vi "Day 3.vi"() -> ()   [LabVIEW 2020]
uses:
  40740d06-73ee-45d0-88f6-0b9eb97e4559.vi
  6b01a3fd-33d4-4bb7-9d17-933a35c8bb1d.vi
  <vilib>/Comparison/Equal/Equal Functor/Equal Functor.lvclass
  <vilib>/regexp/Match Regular Expression.xnode
panel:
  out "sum":i32
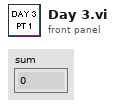
[diagram p1: front panel]
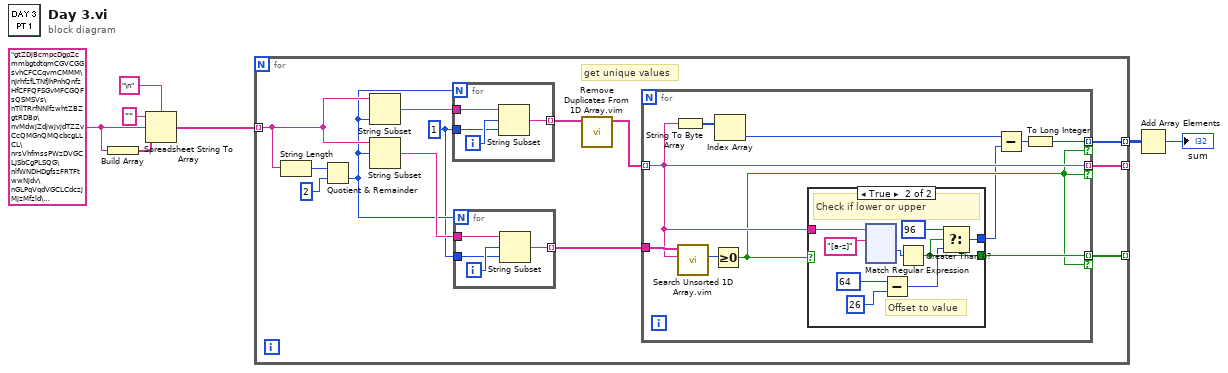
[diagram p0: block diagram]
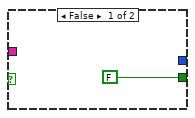
[diagram p2: hidden frame]
diagram:
  w5 = "gtZDjBcmpcDgpZcmmbgtdtqmCGVCGGsvhCFCCqvmCMMM\nJrhfzfLTNfJhPnhQnfzHfCFFQFSGvMFCGQFsQSMSVs\nTllTRrfNNlfzwhtZBZgtRDBp\nvMdwjZdjwjvjdTZZvCcQMGnQMQcbcgLLCL\nrsVhfmssPWzDVGCLJSbCgPLSQG\nlfWNDHDgfszFRTFtwwNjdv\nGLPqVqdVGCLCdczjMjzMfzld\nJnWQvJDmvWBtlMzhrzfHQgcz\ntDtJDDDDtWRRmBwJwWtpPRsGCGScLPGSqspNCS\nChVzZzfNDzNJmBQfjjJfmH\nMrTMPMncGMJvPPvPWTbrMWvgmBgQwgdpwmdpdpjwpHQcdw\nSPvvvbqrFvMvZzJzsFVzVJNV\nmvBbvMFqbMMVVmtCBHpDdDPTDspdNWPDVP\nzjSfftcQtwtSfQSpNDppsNsjPNdRPP\nfgfStJShrgvvCLLv\nGmFnNNwbFFbhQQGQnGwwwfBgnMMqVDBZVVBMfMVzVz\nvWzRRHzTHcgfZDVfBgfH\nSSTvrvRcPpcvjFGwNGbNpbwQwz\nFFgbZZFZgFmpstLgmbtzqNrwVPlMPlSWWrMPNp\nQQhTv..."
  n1 = Build Array(w5) -> (w4:string[])
  n2 = Spreadsheet String To Array(delimiter (Tab)="\n", format string="", spreadsheet string=w5, array type (2D Dbl)=w4) -> (array=w3:string[])
  n3 = for {
    tunnel: w3 -> [w18] mode=indexing
    tunnel: [w14] -> _ mode=indexing
    tunnel: [w13] -> w2 mode=indexing
    tunnel: [w12] -> _ mode=indexing
    w9 = 1 ("length (rest)")
    # "get unique values"
    n4 = String Length(string=w18) -> (length=w20:i32)
    n5 = Quotient & Remainder(x=w20, y=2) -> (floor(x/y)=w10:i32)  [unwired: 1 out]
    n6 = String Subset(string=w18, length (rest)=w10) -> (substring=w17:string)  [unwired: 1 in]
    n7 = String Subset(string=w18, offset (0)=w10) -> (substring=w11:string)  [unwired: 1 in]
    n8 = for {
      N: w10 -> [_]
      tunnel: w17 -> [w162]
      tunnel: [w160] -> w16 mode=indexing
      tunnel: w9 -> [w159]
      i -> [w161]
      n9 = String Subset(string=w162, offset (0)=w161, length (rest)=w159) -> (substring=w160:string)
    }
    n10 = for {
      N: w10 -> [_]
      tunnel: w11 -> [w24]
      tunnel: [w22] -> w8 mode=indexing
      tunnel: w9 -> [w21]
      i -> [w23]
      n11 = String Subset(string=w24, offset (0)=w23, length (rest)=w21) -> (substring=w22:string)
    }
    n12 = call "Remove Duplicates From 1D Array.vim"("array"=w16) -> ("array with duplicates removed"=w15:string[])  [unwired: 10 in]
    n13 = for {
      tunnel: w15 -> [w30] mode=indexing
      tunnel: w8 -> [w34]
      tunnel: [w30] -> w14 mode=indexing if=w28
      tunnel: [w25] -> w13 mode=indexing if=w28
      tunnel: [w29] -> w12 mode=indexing if=w28
      n14 = String To Byte Array(string=w30) -> (unsigned byte array=w32:u8[])
      n15 = call "Search Unsorted 1D Array.vim"("element"=w30, "unsorted 1D array"=w34) -> ("index of element"=w33:i32)  [unwired: 9 in]
      n16 = Greater Or Equal To 0?(x=w33) -> (x >= 0?=w28:bool)
      n17 = Index Array(array=w32) -> (element=w31:u8)  [unwired: 1 in]
      n18 = case shown="True" w28 {
        tunnel: w30 -> [_ w44]
        tunnel: [FALSE w40] -> w29
        tunnel: [_ w38] -> w26
        frame False {
        }
        frame True {
          # "Offset to value"
          # "Check if lower or upper"
          n19 = xnode "Match Regular Expression"("input string"=w44, "regular expression"="[a-z]") -> ("offset past match"=w42:i32)  [unwired: 4 in, 4 out]
          n20 = Subtract(x=u8 64, y=u8 26) -> (x-y=w37:u8)
          n21 = Greater Than 0?(x=w42) -> (x > 0?=w40:bool)
          n22 = Select(t=u8 96, s=w40, f=w37) -> (s? t:f=w38:u8)
        }
      }
      n23 = Subtract(x=w31, y=w26) -> (x-y=w27:u8)
      n24 = To Long Integer(number=w27) -> (32bit integer=w25:i32)
    }
  }
  n25 = Add Array Elements(numeric array=w2) -> (sum=→"sum":i32)
